vi "addArrayDevice.vi"(0 "reference in":refnum<class "Devices Controller.lvclass">, 1 "data in":string[][][](array[string]), 2 "Array":string[](array[string]), 3 "deviceType":T1, 4 "index":i32, 5 "error in (no error)":errorcluster) -> (14 "reference out":refnum<class "Devices Controller.lvclass">, 16 "data out":string[][][](array[string]), 19 "error out":errorcluster)   [LabVIEW 2015, in "Devices Controller.lvclass"]
uses:
  Devices Controller.lvclass
  deviceType.ctl
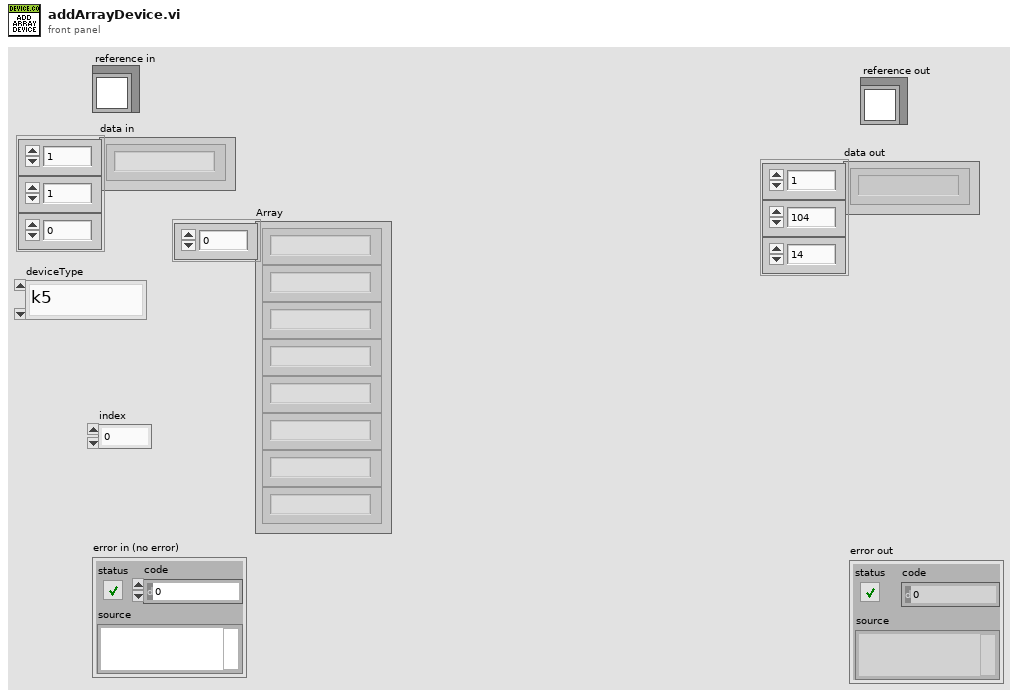
[diagram p1: front panel]
types:
  T1 = typedef "Devices Controller.lvclass/deviceType.ctl" = enum16{"k5", "k4b2", "fitmate", "cpet", "rmr", "bodyBoxPft", "bp", "pp"}
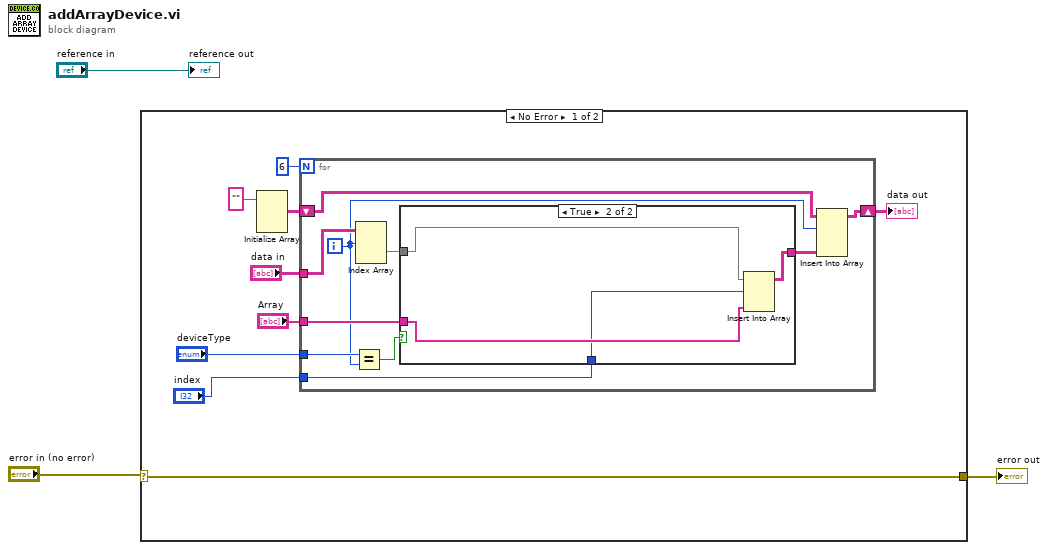
[diagram p0: block diagram]
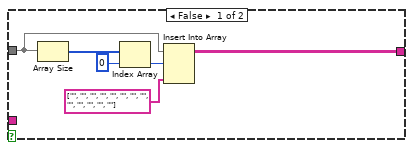
[diagram p2: hidden frame]
diagram:
  n1 = case shown="No Error" "error in (no error)" {
    selector: "error in (no error)" -> [w6 w33]
    tunnel: [w6 w33] -> w1
    frame No Error {
      n2 = Initialize Array("" ("element")) -> (w11:string[][][])  [unwired: 3 in]
      n3 = for {
        N: 6 -> [_]
        tunnel: "deviceType" -> [w15]
        tunnel: "Array" -> [w21]
        shift-right: [w18] -> w7
        shift-left: w11 -> [w20]
        tunnel: "data in" -> [w16]
        tunnel: "index" -> [w13]
        i -> [w14]
        n4 = Equal?(x=w15, y=w14) -> (x = y?=w22:bool)
        n5 = Index Array(array=w16, index (dim 0)=w14) -> (element=w17:string[][])  [unwired: 2 in]
        n6 = case shown="True" w22 {
          tunnel: w17 -> [w28 w32]
          tunnel: w21 -> [_ w31]
          tunnel: [w23 w30] -> w19
          tunnel: w13 -> [_ w29]
          frame False {
            n7 = Array Size(array=w28) -> (size(s)=w26:i32[])
            n8 = Index Array(array=w26, index=0) -> (element=w25:i32)
            n9 = Insert Into Array(array=w28, index (row)=w25, new element=string[] ["", "", "", "", "", "", "", "", "", "", "", "", ""] ("Array 2")) -> (w23:string[][])  [unwired: 1 in]
          }
          frame True {
            n10 = Insert Into Array(array=w32, index (row)=w29, new element=w31) -> (w30:string[][])  [unwired: 1 in]
          }
        }
        n11 = Insert Into Array(array=w20, index (dim 0)=w14, new element=w19) -> (w18:string[][][])  [unwired: 2 in]
      }
      "data out" <- w7
    }
    frame Error {
    }
  }
  "error out" <- w1
  "reference out" <- "reference in"
